vi "inserting_data_database.vi"(0 "connection information":path, 5 "table":string, 7 "Cluster":T1) -> ()   [LabVIEW 2019]
uses:
  <vilib>/addons/database/Connection.llb/DB Tools Open Connec (Path).vi
  <vilib>/addons/database/NI_Database_API.lvlib
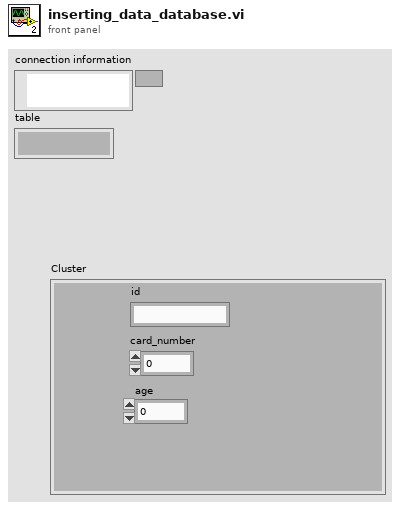
[diagram p1: front panel]
types:
  T1 = cluster{"id":string, "card_number":dbl, "age":dbl}
  T2 = typedef "NI_Database_API.lvlib/Conn ObjectReference.ctl" = refnum<k1>
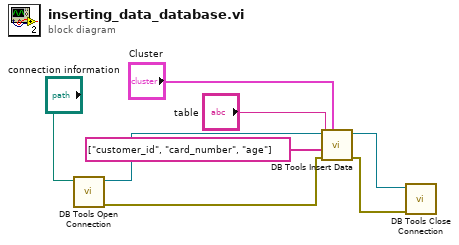
[diagram p0: block diagram]
diagram:
  n1 = call-poly <vilib>:"DB Tools Open Connection.vi"("connection information"="connection information") -> ("error out"=w7:errorcluster, "connection reference"=w5:T2)  [unwired: 7 in]
  n2 = call <vilib>:"DB Tools Insert Data.vi"("data"="Cluster", "error in (no error)"=w7, "columns"=string[] ["customer_id", "card_number", "age"], "table"="table", "connection reference"=w5) -> ("error out"=w6:errorcluster, "connection reference out"=w4:T2)  [unwired: 5 in]
  n3 = call <vilib>:"DB Tools Close Connection.vi"("error in (no error)"=w6, "connection reference"=w4) -> ()  [unwired: 5 in, 1 out]
